vi "Global 1.vi"() -> ()   [LabVIEW 2022 SP3]
panel:
  in  "Array":cluster{"Numeric":dbl, "Numeric 2":dbl}[](array[cluster])
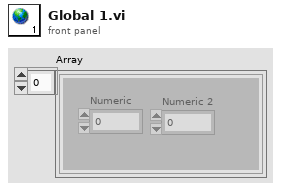
[diagram p1: front panel]
diagram:
